vi "PH_PLH-AccessInformation.contents.vi"   [LabVIEW 2014, in "PH_PLH-AccessInformation.lvlib"]
doc: "This class is forseen to publish the PLH access status.\n\nThis class is part of the PHELIX application layer."
uses:
  PH_PLH-AccessInformation.lvlib
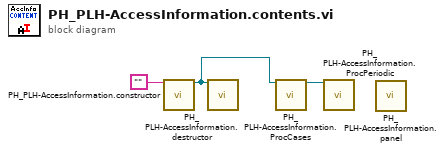
[diagram p0: block diagram]
diagram:
  n1 = call "PH_PLH-AccessInformation.constructor.vi"("name"="") -> ("i ref out"=w1:refnum<vi>)  [unwired: 16 in, 2 out]
  n2 = call "PH_PLH-AccessInformation.destructor.vi"("i ref in"=w1) -> ()  [unwired: 18 in, 1 out]
  n3 = call "PH_PLH-AccessInformation.ProcCases.vi"("i ref in"=w1) -> ("i ref out"=w2:refnum<vi>)  [unwired: 16 in, 2 out]
  n4 = call "PH_PLH-AccessInformation.ProcPeriodic.vi"("i ref in"=w2) -> ()  [unwired: 16 in, 3 out]
  n5 = call "PH_PLH-AccessInformation.panel.vi"() -> ()  [unwired: 19 in, 1 out]
